vi "List tables.vi"(8 "error in (no error)":errorcluster, 11 "database":string) -> (0 "error out":errorcluster, 3 "tables":string[](array[string]))   [LabVIEW 2016, in "database.lvlib"]
uses:
  database.lvlib
  <vilib>/addons/database/Connection.llb/DB Tools Open Connec (String).vi
  <vilib>/addons/database/NI_Database_API.lvlib
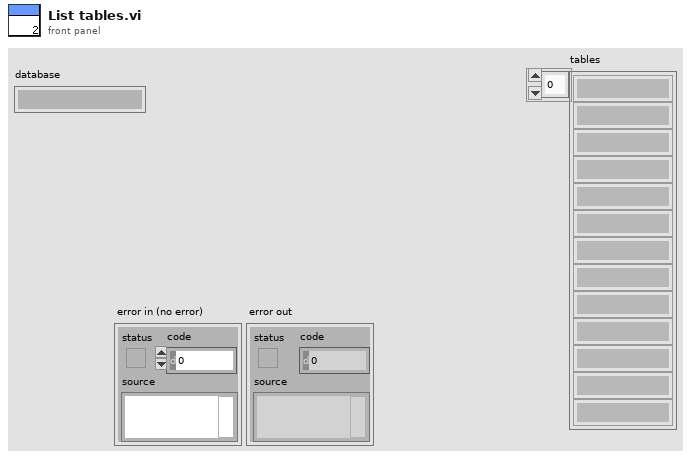
[diagram p1: front panel]
types:
  T1 = typedef "NI_Database_API.lvlib/Conn ObjectReference.ctl" = refnum<k1>
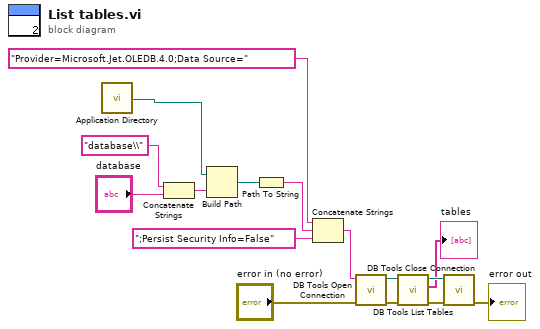
[diagram p0: block diagram]
diagram:
  n1 = call <vilib>:"Application Directory.vi"() -> ("Application Directory"=w1:path)
  n2 = Concatenate Strings("database\\" ("condition"), "database") -> (w4:string)
  n3 = Build Path(base path=w1, name or relative path=w4) -> (appended path=w9:path)
  n4 = Path To String(path=w9) -> (string=w8:string)
  n5 = Concatenate Strings("Provider=Microsoft.Jet.OLEDB.4.0;Data Source=" ("condition"), w8, ";Persist Security Info=False" ("condition")) -> (w6:string)
  n6 = call-poly <vilib>:"DB Tools Open Connection.vi"("error in (no error)"="error in (no error)", "connection information"=w6) -> ("error out"=w14:errorcluster, "connection reference"=w16:T1)  [unwired: 6 in]
  n7 = call <vilib>:"DB Tools List Tables.vi"("error in (no error)"=w14, "connection reference"=w16) -> ("error out"=w13:errorcluster, "tables"=→"tables":string[], "connection reference out"=w15:T1)  [unwired: 3 in]
  n8 = call <vilib>:"DB Tools Close Connection.vi"("error in (no error)"=w13, "connection reference"=w15) -> ("error out"=→"error out":errorcluster)  [unwired: 5 in]
